vi "kalman pv measurement step.vi"(10 "position measurement":i16, 11 "Kalman PV state":T1) -> (3 "kalman pv state out":T1)   [LabVIEW 2010]
uses:
  kalman pv state.ctl
  <vilib>/rvi/FXPMathLib/FxpDiv/XNode/nifxpmath_Div.xnode
  <vilib>/rvi/FXPMathLib/FxpDiv/subVIs/nifxpmath_Div_SimConfig.ctl
  <vilib>/rvi/FXPMathLib/FxpMul/XNode/nifxpmath_Multiplier.xnode
  <vilib>/rvi/FXPMathLib/FxpMul/subVIs/nifxpmath_Mul_SimConfig.ctl
  <vilib>/fxp/LVFixedPointQuantizationPolicyTypeDef.ctl
  <vilib>/fxp/LVFixedPointOverflowPolicyTypeDef.ctl
  <vilib>/rvi/FXPMathLib/FxpSub/XNode/nifxpmath_Sub.xnode
  <vilib>/rvi/FXPMathLib/FxpSub/subVIs/nifxpmath_Sub_SimConfig.ctl
  <vilib>/rvi/FXPMathLib/FxpAdd/XNode/nifxpmath_Add.xnode
  <vilib>/rvi/FXPMathLib/FxpAdd/subVIs/nifxpmath_Add_SimConfig.ctl
  <vilib>/rvi/FXPMathLib/FxpDiv/simVIs/DllFxpDivTemp_sub.vi
  <vilib>/rvi/FXPMathLib/FxpMul/simVIs/DllFxpMulTemp_sub.vi
  <vilib>/rvi/FXPMathLib/FxpSub/simVIs/DllFxpSubTemp_sub.vi
  <vilib>/rvi/FXPMathLib/FxpAdd/simVIs/DllFxpAddTemp_sub.vi
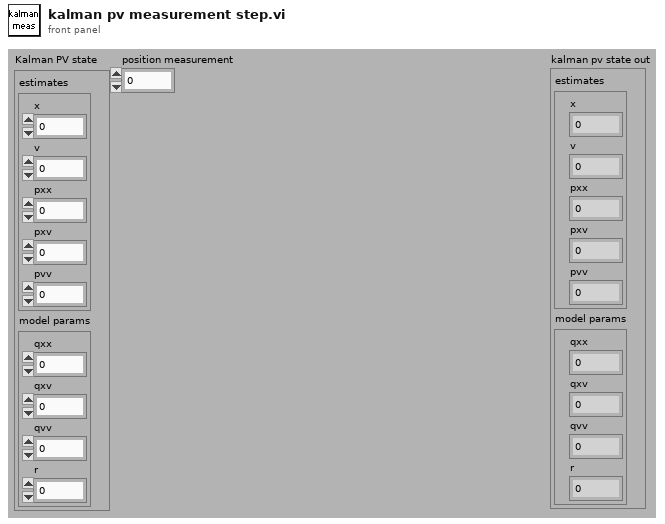
[diagram p1: front panel]
types:
  T1 = typedef "kalman pv state.ctl" = cluster{"estimates":cluster{"x":fxp<+/-,18,16>, "v":fxp<+/-,18,16>, "pxx":u16, "pxv":u16, "pvv":u16}, "model params":cluster{"qxx":u16, "qxv":u16, "qvv":u16, "r":u16}}
  T2 = cluster{"x":fxp<+/-,18,16>, "v":fxp<+/-,18,16>, "pxx":u16, "pxv":u16, "pvv":u16}
  T3 = cluster{"qxx":u16, "qxv":u16, "qvv":u16, "r":u16}
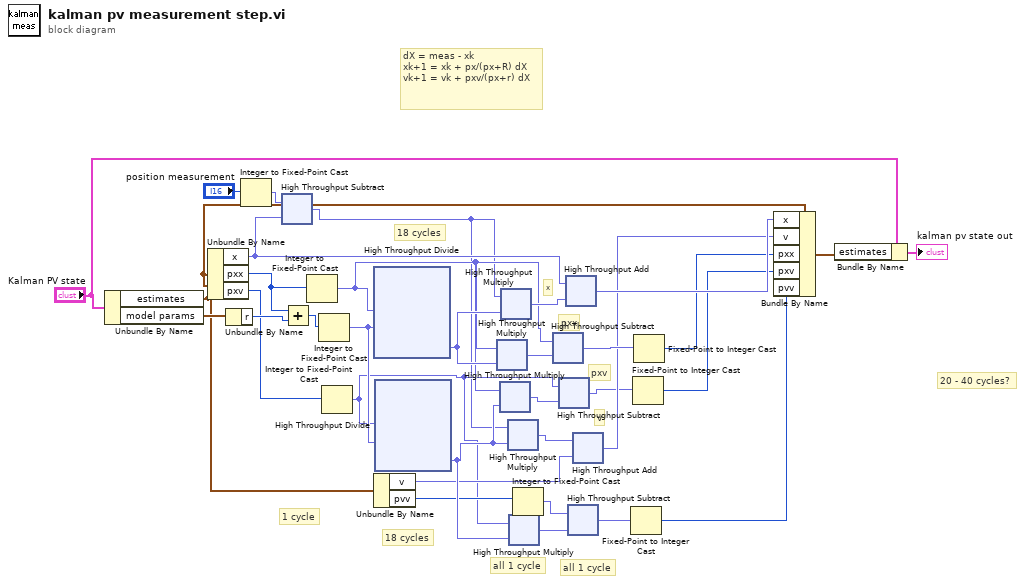
[diagram p0: block diagram]
diagram:
  # "1 cycle"
  # "20 - 40 cycles?"
  # "all 1 cycle"
  # "all 1 cycle"
  # "18 cycles"
  # "18 cycles"
  # "dX = meas - xk\nxk+1 = xk + px/(px+R) dX\nvk+1 = vk + pxv/(px+r) dX"
  # "v"
  # "pxv"
  # "pxx"
  # "x"
  n1 = Unbundle By Name("Kalman PV state") -> ("estimates"=w26:T2, "model params"=w34:T3)
  n2 = Unbundle By Name(w26) -> ("x"=w4:fxp<+/-,18,16>, "pxx"=w31:u16, "pxv"=w30:u16)
  n3 = Unbundle By Name(w34) -> ("r"=w33:u16)
  n4 = Integer to Fixed-Point Cast(integer="position measurement") -> (fixed-point=w2:fxp<+/-,16,16>)  [unwired: 1 in]
  n5 = xnode "High Throughput Subtract"("x"=w2, "y"=w4) -> ("x-y"=w1:fxp<+/-,18,16>)
  n6 = Add(x=w31, y=w33) -> (x+y=w32:u16)
  n7 = Integer to Fixed-Point Cast(integer=w31) -> (fixed-point=w16:fxp<+,16,16>)  [unwired: 1 in]
  n8 = Integer to Fixed-Point Cast(integer=w32) -> (fixed-point=w14:fxp<+,16,16>)  [unwired: 1 in]
  n9 = Integer to Fixed-Point Cast(integer=w30) -> (fixed-point=w5:fxp<+,16,16>)  [unwired: 1 in]
  n10 = xnode "High Throughput Divide"("x"=w16, "y"=w14) -> ("x/y"=w28:fxp<+,16,0>)
  n11 = Unbundle By Name(w26) -> ("v"=w19:fxp<+/-,18,16>, "pvv"=w7:u16)
  n12 = xnode "High Throughput Divide"("x"=w5, "y"=w14) -> ("x/y"=w27:fxp<+,16,0>)
  n13 = xnode "High Throughput Multiply"("x"=w16, "y"=w28) -> ("x*y"=w17:fxp<+/-,16,16>)
  n14 = xnode "High Throughput Multiply"("x"=w16, "y"=w27) -> ("x*y"=w15:fxp<+/-,16,16>)
  n15 = xnode "High Throughput Multiply"("x"=w1, "y"=w28) -> ("x*y"=w29:fxp<+/-,18,16>)
  n16 = xnode "High Throughput Multiply"("x"=w1, "y"=w27) -> ("x*y"=w20:fxp<+/-,18,16>)
  n17 = xnode "High Throughput Multiply"("x"=w5, "y"=w27) -> ("x*y"=w10:fxp<+/-,16,16>)
  n18 = Integer to Fixed-Point Cast(integer=w7) -> (fixed-point=w6:fxp<+,16,16>)  [unwired: 1 in]
  n19 = xnode "High Throughput Subtract"("x"=w16, "y"=w17) -> ("x-y"=w24:fxp<+,16,16>)
  n20 = xnode "High Throughput Subtract"("x"=w5, "y"=w15) -> ("x-y"=w12:fxp<+,16,16>)
  n21 = xnode "High Throughput Add"("x"=w4, "y"=w29) -> ("x+y"=w25:fxp<+/-,18,16>)
  n22 = xnode "High Throughput Subtract"("x"=w6, "y"=w10) -> ("x-y"=w9:fxp<+,16,16>)
  n23 = xnode "High Throughput Add"("x"=w20, "y"=w19) -> ("x+y"=w18:fxp<+/-,18,16>)
  n24 = Fixed-Point to Integer Cast(1:w9) -> (0:w8:u16)
  n25 = Fixed-Point to Integer Cast(1:w12) -> (0:w11:u16)
  n26 = Fixed-Point to Integer Cast(1:w24) -> (0:w13:u16)
  n27 = Bundle By Name(cluster=w26, "x"=w25, "v"=w18, "pxx"=w13, "pxv"=w11, "pvv"=w8) -> (w23:T2)
  n28 = Bundle By Name(cluster="Kalman PV state", "estimates"=w23) -> (→"kalman pv state out":T1)
